vi "fpga_Timestamps_serial_writer.vi"(1 "All Ch Timestamps":T1) -> ()   [LabVIEW 2011]
uses:
  <vilib>/rvi/interface/RandomDataEmulation/niFpgaRandomDataHandleErrors.vi
  <vilib>/rvi/interface/RandomDataEmulation/nirviRandomDataFPGAFIFO.vi
  <vilib>/rvi/DataTransferAndStorage/Container/XNode/niFpgaContainer.xnode
  <vilib>/rvi/interface/RandomDataEmulation/nirviRandomDataFpgaReadWriteTemplate.vi
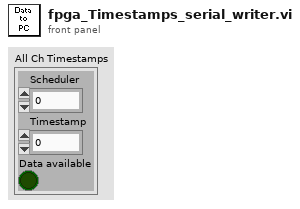
[diagram p1: front panel]
types:
  T1 = cluster{"Scheduler":u8, "Timestamp":u32, "Data available":bool}
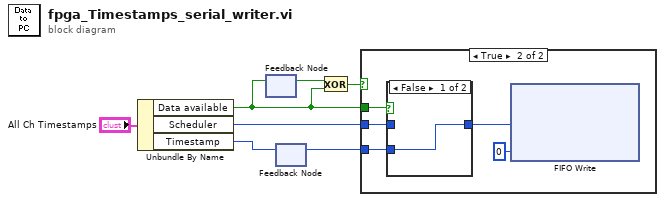
[diagram p0: block diagram]
diagram:
  n1 = Unbundle By Name("All Ch Timestamps") -> ("Data available"=w3:bool, "Scheduler"=w2:u8, "Timestamp"=w1:u32)
  n2 = feedback-in #1(w3) -> ()
  n3 = feedback #1() -> (w6:bool)  [unwired: 1 in]
  n4 = feedback-in #2(w1) -> ()
  n5 = feedback #2() -> (w7:u32)  [unwired: 1 in]
  n6 = Exclusive Or(1:w3, 2:w6) -> (0:w5:bool)
  n7 = case shown="True" w5 {
    tunnel: w2 -> [_ w10]
    tunnel: w7 -> [_ w8]
    tunnel: w3 -> [_ w12]
    frame False {
    }
    frame True {
      n8 = case shown="False" w12 {
        tunnel: w10 -> [_ w14]
        tunnel: [w13 w14] -> w9
        tunnel: w8 -> [w13 _]
        frame False {
        }
        frame True {
        }
      }
      n9 = xnode ("FIFO Write")("Element"=w9, "Timeout"=0) -> ()  [unwired: 1 in, 2 out]
    }
  }
